vi "FuncGaussian2D.vi"(0 "X":dbl[](array[numeric]), 2 "A":dbl[](array[numeric]), 3 "Y":dbl[](array[numeric])) -> (1 "Z":dbl[](array[numeric]))   [LabVIEW 2009]
panel:
  # "x0"
  # "y0"
  # "dx"
  # "dy"
  # "theta"
  # "A"
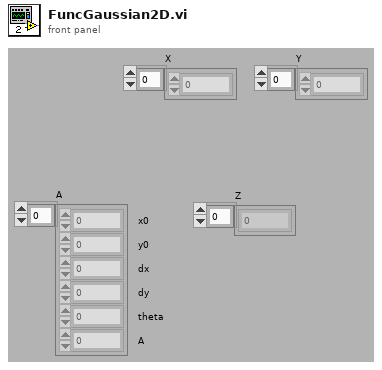
[diagram p1: front panel]
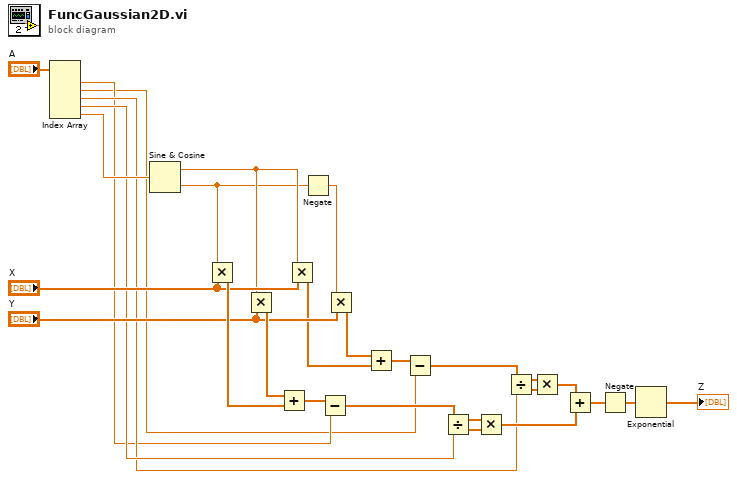
[diagram p0: block diagram]
diagram:
  n1 = Index Array(array="A") -> (element #1=w5:dbl, element #2=w4:dbl, element #3=w6:dbl, element #4=w7:dbl, element #5=w25:dbl)  [unwired: 5 in]
  n2 = Sine & Cosine(0:w25) -> (1:w21:dbl, 2:w19:dbl)
  n3 = Multiply(x=w19, y="X") -> (x*y=w23:dbl[])
  n4 = Multiply(x=w21, y="Y") -> (x*y=w24:dbl[])
  n5 = Add(x=w24, y=w23) -> (x+y=w8:dbl[])
  n6 = Multiply(x=w21, y="X") -> (x*y=w17:dbl[])
  n7 = Negate(x=w19) -> (-x=w18:dbl)
  n8 = Subtract(x=w8, y=w5) -> (x-y=w9:dbl[])
  n9 = Multiply(x=w18, y="Y") -> (x*y=w16:dbl[])
  n10 = Add(x=w16, y=w17) -> (x+y=w15:dbl[])
  n11 = Subtract(x=w15, y=w4) -> (x-y=w10:dbl[])
  n12 = Divide(x=w9, y=w7) -> (x/y=w14:dbl[])
  n13 = Multiply(x=w14, y=w14) -> (x*y=w11:dbl[])
  n14 = Divide(x=w10, y=w6) -> (x/y=w13:dbl[])
  n15 = Multiply(x=w13, y=w13) -> (x*y=w12:dbl[])
  n16 = Add(x=w12, y=w11) -> (x+y=w3:dbl[])
  n17 = Negate(x=w3) -> (-x=w2:dbl[])
  n18 = Exponential(1:w2) -> (0:→"Z":dbl[])
